vi "Test_distance_to_position.vi"(2 "Channel":T1={"X Pos (mm)"=-1.904501, "Y Pos (mm)"=-0.42059234, "Z Pos (mm)"=-0.07494753} {"Y Pos (mm)" format="%.3f"; "Z Pos (mm)" format="%.3f"; "X Pos (mm)" format="%.3f"}, 3 "Current position":T1={"X Pos (mm)"=0.15566698, "Y Pos (mm)"=-0.2807253, "Z Pos (mm)"=-0.118062034} {"Y Pos (mm)" format="%.3f"; "Z Pos (mm)" format="%.3f"; "X Pos (mm)" format="%.3f"}) -> (0 "All out of range?":bool, 1 "Output distance":T1={"X Pos (mm)"=-1.904501, "Y Pos (mm)"=-0.42059234, "Z Pos (mm)"=-0.07494753} {"Y Pos (mm)" format="%.3f"; "Z Pos (mm)" format="%.3f"; "X Pos (mm)" format="%.3f"})   [LabVIEW 2014]
panel:
  in  "Distance":T1={"X Pos (mm)"=-1.904501, "Y Pos (mm)"=-0.42059234, "Z Pos (mm)"=-0.07494753} {"Y Pos (mm)" format="%.3f"; "Z Pos (mm)" format="%.3f"; "X Pos (mm)" format="%.3f"}
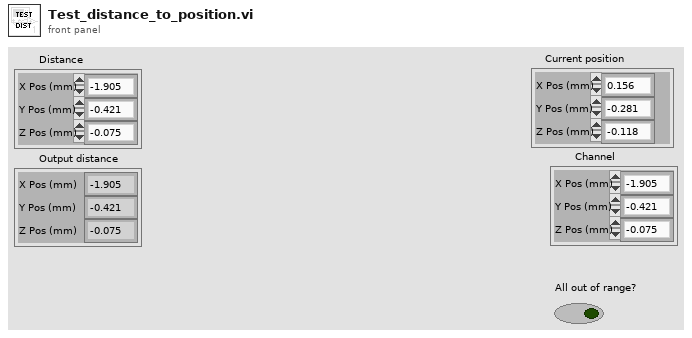
[diagram p1: front panel]
types:
  T1 = cluster{"X Pos (mm)":sgl, "Y Pos (mm)":sgl, "Z Pos (mm)":sgl}
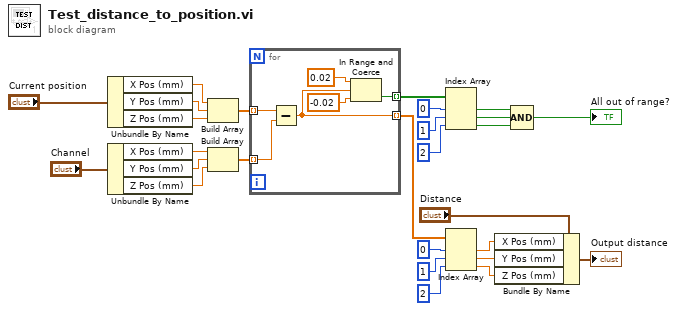
[diagram p0: block diagram]
diagram:
  n1 = Unbundle By Name("Current position") -> ("X Pos (mm)"=w24:sgl, "Y Pos (mm)"=w23:sgl, "Z Pos (mm)"=w22:sgl)
  n2 = Unbundle By Name("Channel") -> ("X Pos (mm)"=w21:sgl, "Y Pos (mm)"=w20:sgl, "Z Pos (mm)"=w19:sgl)
  n3 = Build Array(w24, w23, w22) -> (w18:sgl[])
  n4 = Build Array(w21, w20, w19) -> (w17:sgl[])
  n5 = for {
    tunnel: w18 -> [w33] mode=indexing
    tunnel: w17 -> [w32] mode=indexing
    tunnel: [w29] -> w16 mode=indexing
    tunnel: [w28] -> w6 mode=indexing
    n6 = Subtract(x=w33, y=w32) -> (x-y=w28:sgl)
    n7 = In Range and Coerce(upper limit=0.02, x=w28, lower limit=-0.02) -> (In Range?=w29:bool)  [unwired: 1 out]
  }
  n8 = Index Array(array=w16, index #1=0, index #2=1, index #3=2) -> (element #1=w10:bool, element #2=w12:bool, element #3=w11:bool)
  n9 = Index Array(array=w6, index #1=0, index #2=1, index #3=2) -> (element #1=w5:sgl, element #2=w4:sgl, element #3=w3:sgl)
  n10 = Bundle By Name(cluster="Distance", "X Pos (mm)"=w5, "Y Pos (mm)"=w4, "Z Pos (mm)"=w3) -> (→"Output distance":T1)
  n11 = Compound Arithmetic op=AND(w10, w12, w11) -> (→"All out of range?":bool)
